vi "Esempio.vi"() -> ()   [LabVIEW 2016]
panel:
  in  "stop":bool
  in  "Errori max 2":dbl
  in  "COM WT1600":string
  in  "error inWT1600":errorcluster
  in  "termination char\n(0xA = '\\n' = LF)":u8=10 format="%.0x"
  in  "Wiring A (0: 1P2W)":u16(ring) items=["1P2W", "1P3W", "3P3W", "3P4W", "3V3A"]
  in  "Wiring B (0: 1P2W)":u16(ring) items=["1P2W", "1P3W", "3P3W", "3P4W", "3V3A", "NONE"]
  in  "Wiring C (0: 1P2W)":u16(ring) items=["1P2W", "1P3W", "3P3W", "3P4W", "3V3A", "NONE"]
  in  "Number of Item (15)":u16=15 min=1 max=255 step=1
  in  "Preset (2: Preset 2)":u16(ring)=2 items=["", "Preset1", "Preset2", "Preset3", "Preset4"]
  out "Measure":dbl[](array[numeric]) format="%^.4e"
  in  "Leggi":bool
  in  "String1":string=":NUM:NORM:NUM 4;ITEM1 IMN,1;ITEM2 IMN,2;ITEM3 IMN,3;ITEM4 IMN,4; VAL?;"
  in  "String2":string=":NUM:NORM:NUM 4;ITEM1 IMN,1;ITEM2 IMN,2;ITEM3 IMN,3;ITEM4 IMN,4; VAL?;"
  in  "String3":string=":NUM:NORM:NUM 4;ITEM1 IMN,1;ITEM2 IMN,2;ITEM3 IMN,3;ITEM4 IMN,4; VAL?;"
  in  "String5":string=":NUM:NORM:NUM 4;ITEM1 IMN,1;ITEM2 IMN,2;ITEM3 IMN,3;ITEM4 IMN,4; VAL?;"
  in  "String4":string=":NUM:NORM:NUM 4;ITEM1 IMN,1;ITEM2 IMN,2;ITEM3 IMN,3;ITEM4 IMN,4; VAL?;"
  in  "Abilita preset 2":bool
  out "Errori WT1600":i8
  out "WT1600":bool
  out "Simulazione":bool
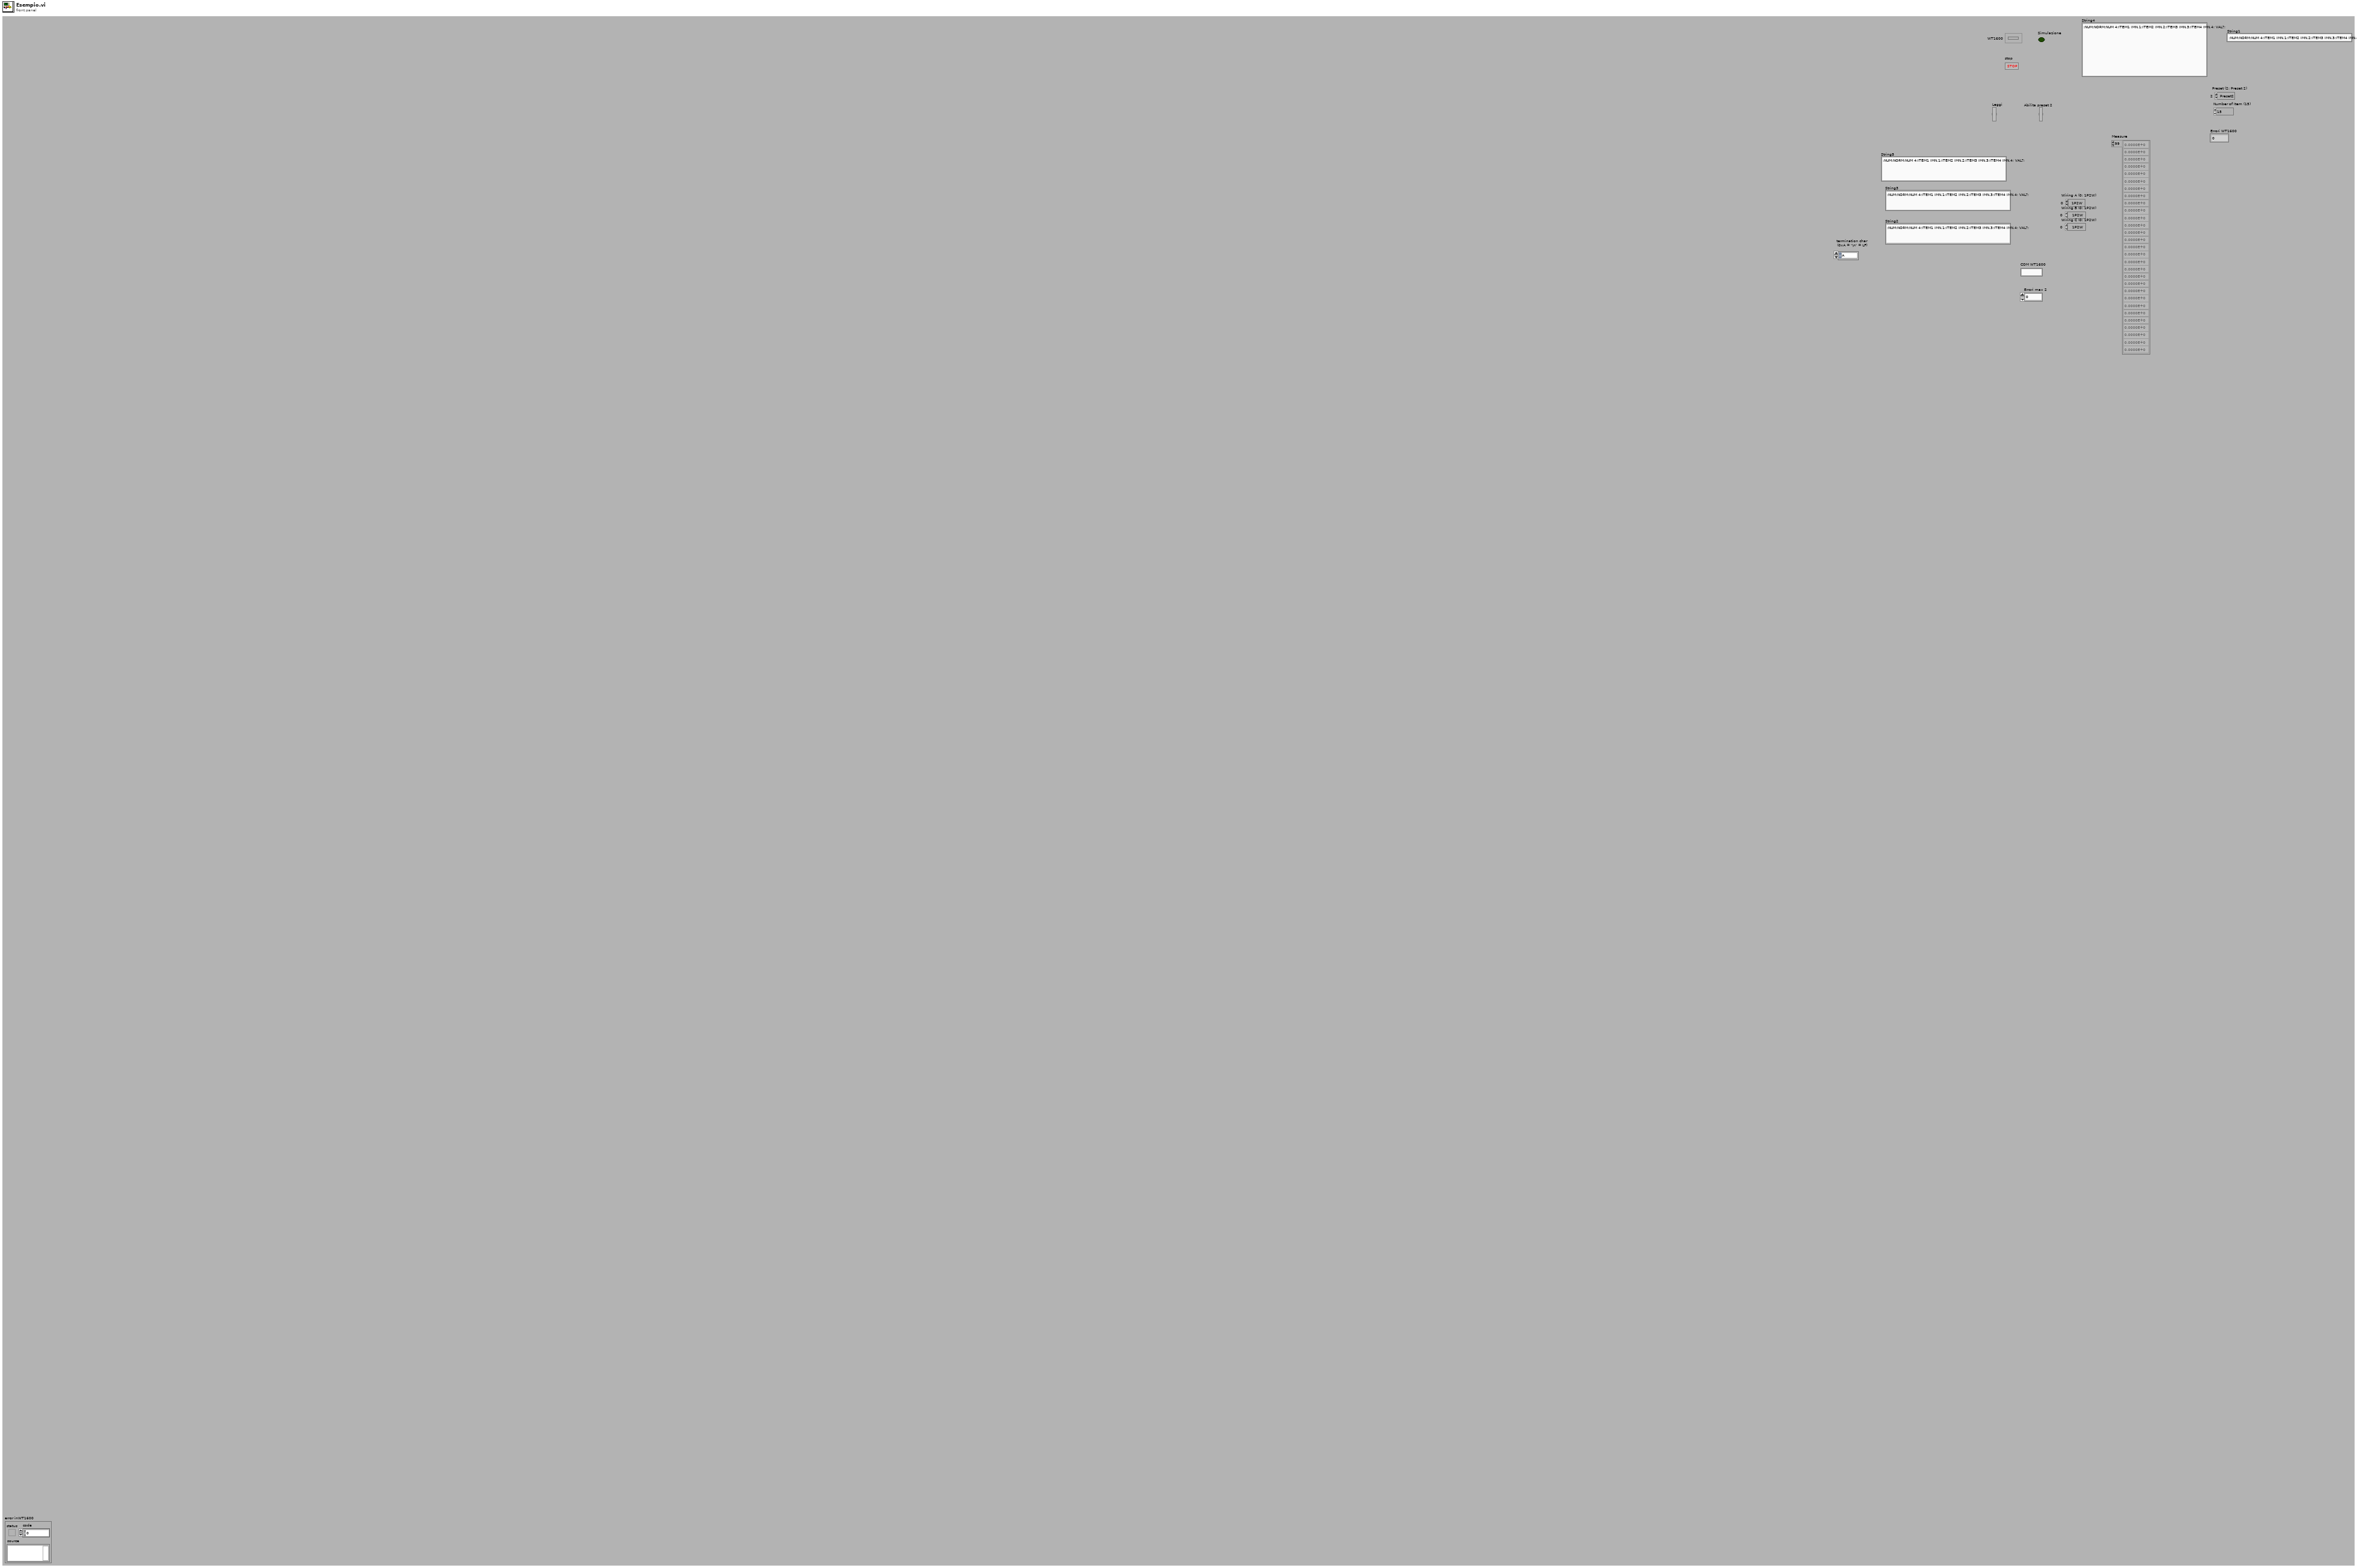
[diagram p1: front panel]
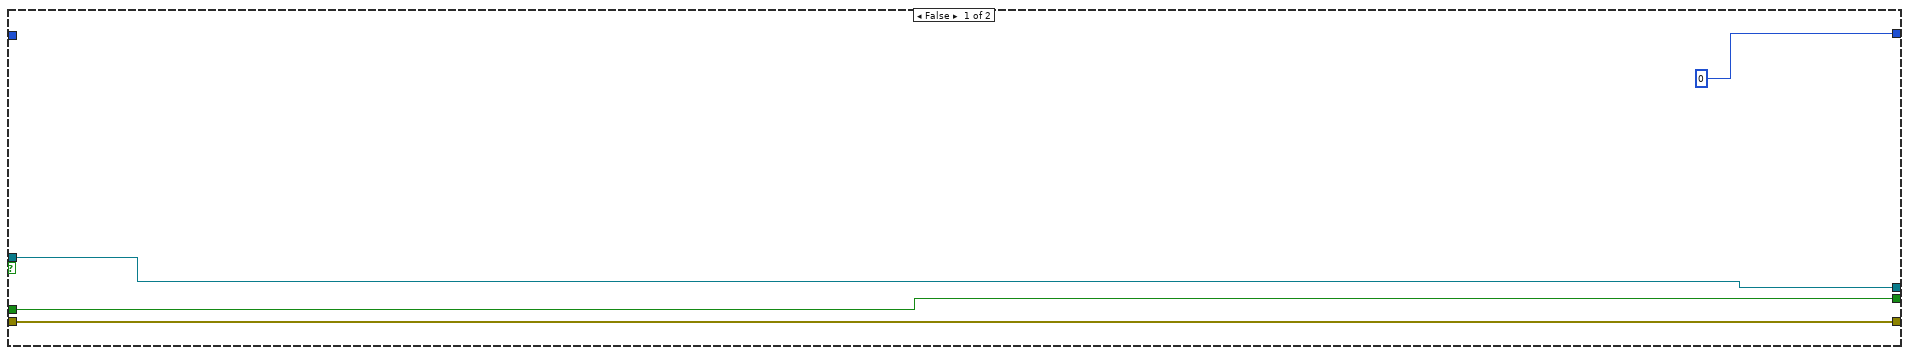
[diagram p2: hidden frame]
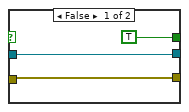
[diagram p7: hidden frame]
diagram:
  n1 = while {
    shift-right: [w15] -> w2
    shift-left: _ -> [w16]
    shift-right: [w14] -> w1
    shift-left: "error inWT1600" -> [w13]
    shift-right: [w12] -> _
    shift-left: FALSE -> [w17]
    shift-right: [w8] -> _
    shift-left: 0 -> [w9]
    stop <- "stop" stop-if-true
    n2 = local read "Simulazione"() -> (w11:bool)
    n3 = Not(x=w11) -> (.not. x?=w10:bool)
    n4 = case shown="True" w10 {
      tunnel: w17 -> [w19 w35]
      tunnel: w16 -> [w20 w48]
      tunnel: [w20 w47] -> w15
      tunnel: [w21 w46] -> w14
      tunnel: w13 -> [w21 w45]
      tunnel: [w19 w44] -> w12
      tunnel: w9 -> [_ w31]
      tunnel: [0 w30] -> w8
      frame False {
      }
      frame True {
        n5 = case shown="False" w35 {
          tunnel: [w83 w108] -> w40
          tunnel: [w84 w109] -> w41
          tunnel: w45 -> [_ w109]
          tunnel: w48 -> [_ w108]
          frame False {
            w104 = TRUE
            w105 = TRUE
            # "Config\nCurrent"
            # "Config\nVoltage"
            # "Initialize"
            n6 = local read "COM WT1600"() -> (w94:string)
            n7 = call "OpenCOM.vi"("VISA resource name"=w94, "baud rate (9600)"=19200, "data bits"=8, "parity"=0, "stop bits"=10, "flow control"=0, "termination char\n(0xA = '\\n' = LF)"="termination char\n(0xA = '\\n' = LF)", "timeout(ms) solitamente 50ms"=2000, "End Write termination character?"=w104, "End read on termination character?"=w104) -> ("VISA resource name out"=w103:refnum<visa-resource-name>, "error out"=w102:errorcluster)  [unwired: 16 in]
            n8 = call "WT1600(Init).vi"("VISA session 2"=w103, "ID Query (T: Check)"=w105, "Reset (T: Reset)"=w105, "error in (no error)"=w102) -> ("VISA session"=w107:refnum<visa-resource-name>, "error out"=w106:errorcluster)  [unwired: 10 in]
            n9 = call "YKWT1600 Config Voltage.vi"("VISA session"=w107, "V Range (12: 1000)"=11, "error in (no error)"=w106) -> ("dup VISA session"=w92:refnum<visa-resource-name>, "error out"=w93:errorcluster)  [unwired: 11 in]
            n10 = call "YKWT1600 Config Current.vi"("VISA session"=w92, "A Range (9: 5A)"=5, "error in (no error)"=w93) -> ("dup VISA session"=w89:refnum<visa-resource-name>, "error out"=w88:errorcluster)  [unwired: 11 in]
            n11 = call "YKWT1600 Config Wiring.vi"("VISA session"=w89, "Wiring A (0: 1P2W)"="Wiring A (0: 1P2W)", "Wiring B (0: 1P2W)"="Wiring B (0: 1P2W)", "Wiring C (0: 1P2W)"="Wiring C (0: 1P2W)", "error in (no error)"=w88) -> ("dup VISA session"=w83:refnum<visa-resource-name>, "error out"=w84:errorcluster)  [unwired: 9 in]
          }
          frame True {
          }
        }
        n12 = Less Or Equal?(x=w31, y=14) -> (x <= y?=w33:bool)
        n13 = And(x=w33, y=w35) -> (x .and. y?=w34:bool)
        n14 = Or(x=w34, y="Abilita preset 2") -> (x .or. y?=w37:bool)
        n15 = case shown="True" w37 {
          tunnel: w40 -> [w50 w54]
          tunnel: w41 -> [w49 w51]
          tunnel: [w50 w53] -> w39
          tunnel: [w49 w52] -> w38
          frame False {
          }
          frame True {
            n16 = case shown="No Error" w51 {
              tunnel: w54 -> [w58 w73]
              tunnel: w51 -> [w57 w72]
              tunnel: [w56 w73] -> w53
              tunnel: [w55 w72] -> w52
              frame No Error {
                n17 = VISA Write(VISA resource name=w58, write buffer="String1", error in (no error)=w57) -> (VISA resource name out=w68:refnum<visa-resource-name>, error out=w67:errorcluster)  [unwired: 1 out]
                n18 = VISA Write(VISA resource name=w68, write buffer="String2", error in (no error)=w67) -> (VISA resource name out=w66:refnum<visa-resource-name>, error out=w65:errorcluster)  [unwired: 1 out]
                n19 = VISA Write(VISA resource name=w66, write buffer="String3", error in (no error)=w65) -> (VISA resource name out=w62:refnum<visa-resource-name>, error out=w61:errorcluster)  [unwired: 1 out]
                n20 = VISA Write(VISA resource name=w62, write buffer="String5", error in (no error)=w61) -> (VISA resource name out=w60:refnum<visa-resource-name>, error out=w59:errorcluster)  [unwired: 1 out]
                n21 = VISA Write(VISA resource name=w60, write buffer="String4", error in (no error)=w59) -> (VISA resource name out=w56:refnum<visa-resource-name>, error out=w55:errorcluster)  [unwired: 1 out]
              }
              frame Error {
              }
            }
          }
        }
        n22 = case shown="True" "Leggi" {
          tunnel: w39 -> [w75 w82]
          tunnel: w38 -> [w74 w81]
          tunnel: [w75 w80] -> w23
          tunnel: [w74 w79] -> w22
          tunnel: "Number of Item (15)" -> [_ w77]
          frame False {
          }
          frame True {
            n23 = call "YKWT1600 Read Preset Numeric Normal.vi"("VISA session"=w82, "Preset (2: Preset 2)"="Preset (2: Preset 2)", "Number of Item (15)"=w77, "error in (no error)"=w81) -> ("dup VISA session"=w80:refnum<visa-resource-name>, "Measure"=→"Measure":dbl[], "error out"=w79:errorcluster)  [unwired: 8 in, 1 out]
          }
        }
        n24 = local read "Errori max 2"() -> (w24:dbl)
        n25 = local read "Errori WT1600"() -> (w26:i8)
        n26 = call "Com Errori.vi"("VISA session"=w23, "Errori in"=w26, "Max Errori"=w24, "error in (no error)"=w22) -> ("dup VISA session"=w29:refnum<visa-resource-name>, "Errori out"=w25:i64, "Chiudi com"=w27:bool, "error out"=w28:errorcluster)  [unwired: 20 in]
        n27 = local write "Errori WT1600"(w25) -> ()
        n28 = case shown="True" w27 {
          selector: w27 -> [_ w114]
          tunnel: w28 -> [w111 w118]
          tunnel: w29 -> [w112 w117]
          tunnel: [w111 w116] -> w46
          tunnel: [w112 w115] -> w47
          tunnel: [TRUE w113] -> w44
          frame False {
          }
          frame True {
            n29 = call <instrlib>:"YKWT1600 Error Query (multiple).vi"("VISA session"=w117, "error in (no error)"=w118) -> ("dup VISA session"=w115:refnum<visa-resource-name>, "error out"=w119:errorcluster)  [unwired: 10 in, 2 out]
            n30 = call "YKWT1600 Close.vi"("VISA session"=w115, "error in (no error)"=w119) -> ("error out"=w116:errorcluster)  [unwired: 13 in]
            n31 = Not(x=w114) -> (.not. x?=w113:bool)
          }
        }
        n32 = Increment(x=w31) -> (x+1=w30:i32)
      }
    }
    "WT1600" <- w12
    n33 = Wait Until Next ms Multiple(millisecond multiple=200) -> ()  [unwired: 1 out]
  }
  n34 = VISA Close(VISA resource name=w2, error in (no error)=w1) -> ()  [unwired: 1 out]
